vi "Turning.vi"(0 "Turn Rate":dbl) -> (1 "Left Motor":dbl, 2 "Right Motor":dbl)   [LabVIEW 2015]
panel:
  in  "Min Motor Value":dbl=0.08
  # "Negative is turning left (as per the gyro)"
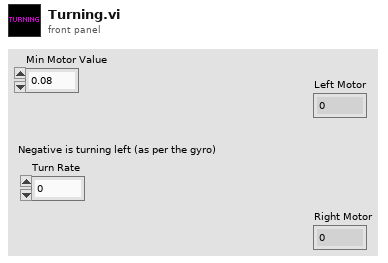
[diagram p1: front panel]
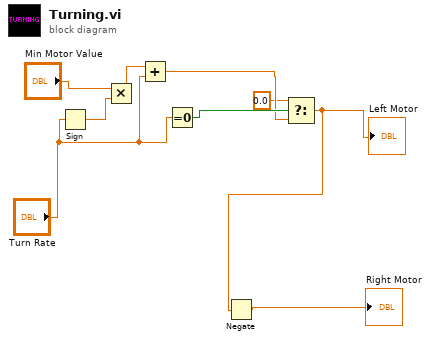
[diagram p0: block diagram]
diagram:
  n1 = Sign(1:"Turn Rate") -> (0:w7:dbl)
  n2 = Multiply(x="Min Motor Value", y=w7) -> (x*y=w8:dbl)
  n3 = Add(x=w8, y="Turn Rate") -> (x+y=w5:dbl)
  n4 = Equal To 0?(x="Turn Rate") -> (x = 0?=w9:bool)
  n5 = Select(t=0.0, s=w9, f=w5) -> (s? t:f=w2:dbl)
  "Left Motor" <- w2
  n6 = Negate(x=w2) -> (-x=→"Right Motor":dbl)
